vi "uTTA_SetCALSamplerate.vi"(8 "error in":errorcluster, 10 "Calibration SampleRate(ms)":u16, 11 "VISA Refnum in":refnum<visa-resource-name>) -> (0 "error out":errorcluster, 3 "VISA Refnum out":refnum<visa-resource-name>, 4 "CAL SampleRate(ms)":u32, 7 "Received":string)   [LabVIEW 2021]
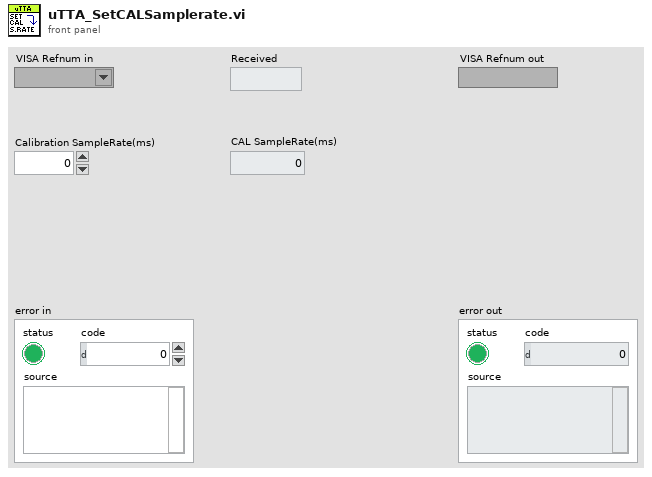
[diagram p1: front panel]
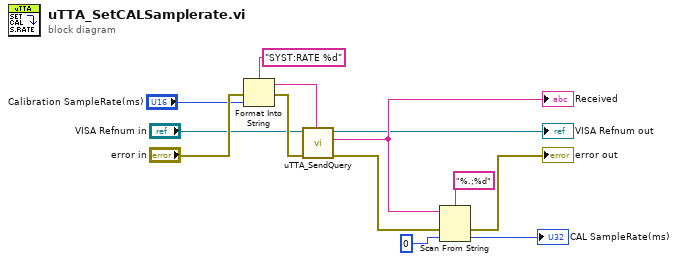
[diagram p0: block diagram]
diagram:
  n1 = Format Into String(format string="SYST:RATE %d", error in="error in", "Calibration SampleRate(ms)") -> (resulting string=w6:string, error out=w8:errorcluster)  [unwired: 1 in]
  n2 = call "uTTA_SendQuery.vi"("Send String"=w6, "error in (no error)"=w8, "VISA Refnum in"="VISA Refnum in") -> ("error out"=w11:errorcluster, "Received"=w9:string, "VISA Refnum out"=→"VISA Refnum out":refnum<visa-resource-name>)  [unwired: 6 in]
  "Received" <- w9
  n3 = Scan From String(format string="%.;%d", input string=w9, error in=w11, default 1=u32 0 ("default value 1")) -> (error out=→"error out":errorcluster, output 1=→"CAL SampleRate(ms)":u32)  [unwired: 1 in, 2 out]
